vi "set_timing_source.vi"(8 "error in (no error)":errorcluster, 10 "timing source":tag, 11 "DAQmxWriteSignals.lvclass in":refnum<class "SignalWriterDL090202DAQmx.lvclass">) -> (0 "error out":errorcluster, 3 "DAQmxWriteSignals.lvclass out":refnum<class "SignalWriterDL090202DAQmx.lvclass">)   [LabVIEW 2010, in "SignalWriterDL090202DAQmx.lvclass"]
uses:
  SignalWriterDL090202DAQmx.lvclass
  SignalWriterDL090202DAQmx.lvclass/SignalWriterDL090202DAQmx.ctl
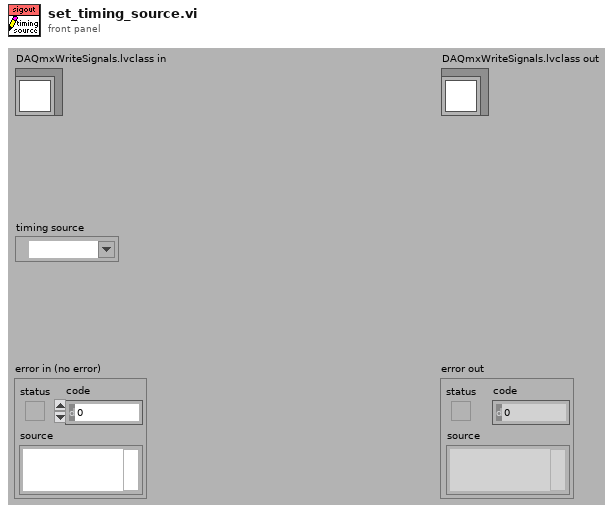
[diagram p1: front panel]
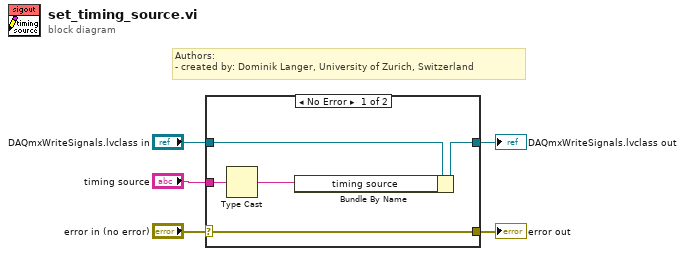
[diagram p0: block diagram]
diagram:
  # "Authors: \n- created by: Dominik Langer, University of Zurich, Switzerland"
  n1 = case shown="No Error" "error in (no error)" {
    selector: "error in (no error)" -> [w10 w11]
    tunnel: [w10 w11] -> w4
    tunnel: [w8 w12] -> w2
    tunnel: "DAQmxWriteSignals.lvclass in" -> [w9 w12]
    tunnel: "timing source" -> [w7 _]
    frame No Error {
      n2 = Type Cast(x=w7) -> (*(type *) &x=w6:string)  [unwired: 1 out]
      n3 = Bundle By Name(cluster=w9, "timing source"=w6) -> (w8:refnum<class "SignalWriterDL090202DAQmx.lvclass">)
    }
    frame Error {
    }
  }
  "error out" <- w4
  "DAQmxWriteSignals.lvclass out" <- w2
